vi "Initialize Camera.vi"(8 "error in (no error)":errorcluster, 11 "CCDCamera in":refnum<class "CCDCamera.lvclass">) -> (0 "error out":errorcluster, 3 "CCDCamera out":refnum<class "CCDCamera.lvclass">)   [LabVIEW 2018, in "CCDCamera.lvclass"]
uses:
  CCDCamera.lvclass
  C:/Users/observer/Desktop/SPARC4_ACS/Simulated_CCD_Camera/Simulated_CCD_Camera.lvclass
  Simulated_CCD_Camera/Simulated_CCD_Camera.lvclass/Simulated_CCD_Camera.ctl
  Simulated_CCD_Camera/Simulated_CCD_Camera.lvclass
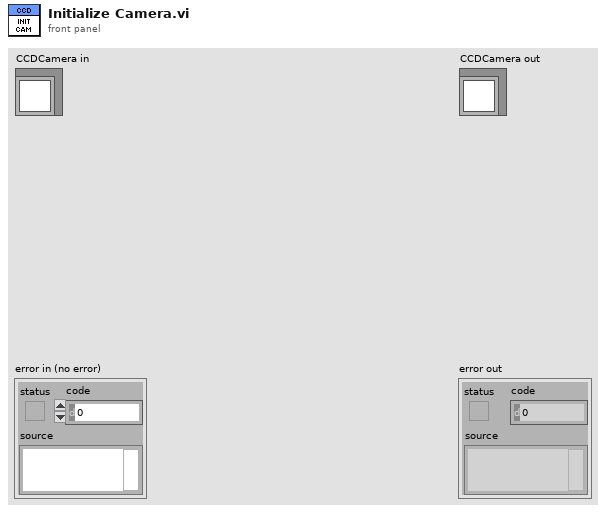
[diagram p1: front panel]
types:
  T1 = cluster{"Acquiring":bool, "Current exptime":sgl, "STATUS":string, "Exposures Done":u16}
  T2 = cluster{"Initialization":bool, "Serial Number":u16}
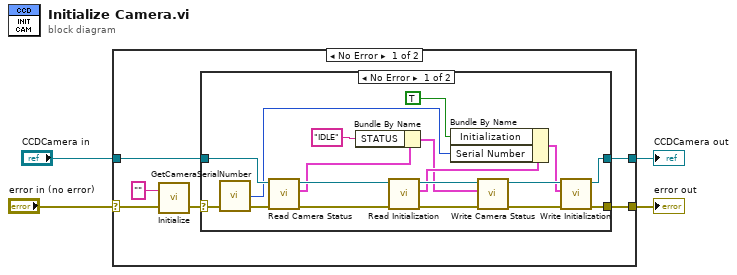
[diagram p0: block diagram]
diagram:
  n1 = case shown="No Error" "error in (no error)" {
    selector: "error in (no error)" -> [w9 w32]
    tunnel: [w7 w32] -> w1
    tunnel: [w8 w31] -> w2
    tunnel: "CCDCamera in" -> [w6 w31]
    frame No Error {
      n2 = call <userlib>:"Initialize.vi"("error in (no error)"=w9, "directory (\"\")"="" ("directory (\"\")")) -> ("error out"=w10:errorcluster)  [unwired: 1 out]
      n3 = case shown="No Error" w10 {
        selector: w10 -> [w27 w29]
        tunnel: w6 -> [w17 w30]
        tunnel: [w21 w30] -> w8
        tunnel: [w22 w29] -> w7
        frame No Error {
          n4 = call <userlib>:"GetCameraSerialNumber.vi"("error in (no error)"=w27) -> ("error out"=w26:errorcluster, "number"=w14:i32)  [unwired: 2 in, 1 out]
          n5 = call "Read Camera Status.vi"("error in (no error)"=w26, "CCDCamera in"=w17) -> ("error out"=w25:errorcluster, "Camera Status"=w16:T1, "CCDCamera out"=w18:refnum<class "CCDCamera.lvclass">)  [unwired: 7 in]
          n6 = Bundle By Name(cluster=w16, "STATUS"="IDLE" ("Camera Status.STATUS")) -> (w11:T1)
          n7 = call "Read Initialization.vi"("error in (no error)"=w25, "CCDCamera in"=w18) -> ("error out"=w24:errorcluster, "Initialization"=w15:T2, "CCDCamera out"=w19:refnum<class "CCDCamera.lvclass">)  [unwired: 7 in]
          n8 = Bundle By Name(cluster=w15, "Initialization"=TRUE, "Serial Number"=w14) -> (w12:T2)
          n9 = call "Write Camera Status.vi"("error in (no error)"=w24, "Camera Status"=w11, "CCDCamera in"=w19) -> ("error out"=w23:errorcluster, "CCDCamera out"=w20:refnum<class "CCDCamera.lvclass">)  [unwired: 7 in]
          n10 = call "Write Initialization.vi"("error in (no error)"=w23, "Initialization"=w12, "CCDCamera in"=w20) -> ("error out"=w22:errorcluster, "CCDCamera out"=w21:refnum<class "CCDCamera.lvclass">)  [unwired: 7 in]
        }
        frame Error {
        }
      }
    }
    frame Error {
    }
  }
  "error out" <- w1
  "CCDCamera out" <- w2
